vi "cargarDatoProducto.vi"(11 "IndiceAUltimoValor\nAgregadoEnLaTabla":i32=1) -> ()   [LabVIEW 2014]
uses:
  claseProducto/claseProducto.lvclass
panel:
  out "dataReading":T1
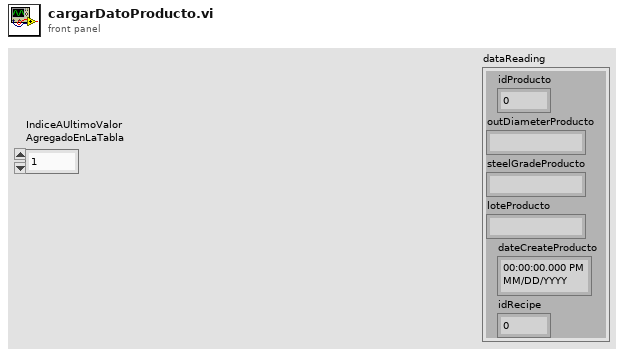
[diagram p1: front panel]
types:
  T1 = cluster{"idProducto":dbl, "outDiameterProducto":string, "steelGradeProducto":string, "loteProducto":string, "dateCreateProducto":timestamp, "idRecipe":dbl}
  T2 = cluster{i32, "od":string, "steelGrade":string, "lote":string, "seconds since 1Jan1904":timestamp, "idRecipe":dbl}
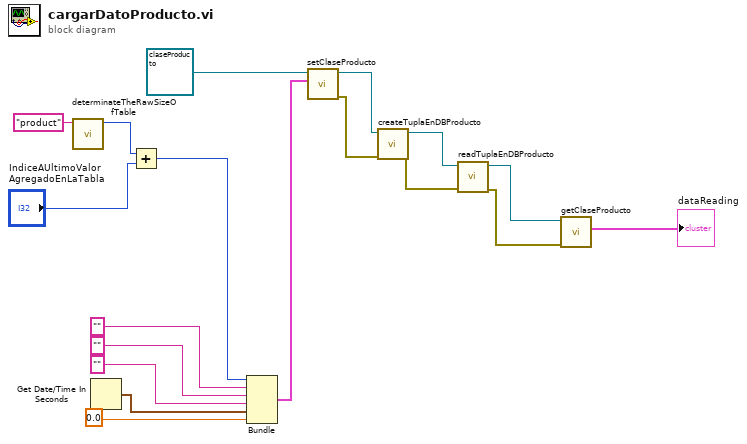
[diagram p0: block diagram]
diagram:
  n1 = call "determinateTheRawSizeOfTable.vi"("tableName"="product") -> ("sizeOfTableInNumberRaw"=w2:i32)  [unwired: 8 in, 1 out]
  n2 = Get Date/Time In Seconds() -> (seconds since 1Jan1904=w13:timestamp)
  n3 = Add(x=w2, y="IndiceAUltimoValor\nAgregadoEnLaTabla") -> (x+y=w4:i32)
  n4 = Bundle(w4, "od"="", "steelGrade"="", "lote"="", "seconds since 1Jan1904"=w13, "idRecipe"=0.0) -> (w14:T2)  [unwired: 1 in]
  n5 = call "setClaseProducto.vi"("Cluster of class private data"=w14, "claseProducto in"=refnum<class "claseProducto.lvclass"> refnum ("claseProducto.lvclass")) -> ("error out"=w11:errorcluster, "claseProducto out"=w12:refnum<class "claseProducto.lvclass">)  [unwired: 6 in]
  n6 = call "createTuplaEnDBProducto.vi"("error in"=w11, "claseProducto in"=w12) -> ("error out"=w9:errorcluster, "claseProducto out"=w10:refnum<class "claseProducto.lvclass">)  [unwired: 8 in]
  n7 = call "readTuplaEnDBProducto.vi"("error in"=w9, "claseProducto in"=w10) -> ("error out"=w7:errorcluster, "claseProducto out"=w8:refnum<class "claseProducto.lvclass">)  [unwired: 8 in]
  n8 = call "getClaseProducto.vi"("claseProducto.lvclass"=w8, "error in"=w7) -> ("dataReading"=→"dataReading":T1)  [unwired: 6 in, 2 out]
